vi "Periodic Tasks.vi"(11 "Initalizer":bool) -> ()   [LabVIEW 2014]
doc: "This VI runs in parallel to other tasks. It can contain as many user-defined periodic loops as you need. These can carry out PID or other sorts of timed response."
uses:
  <vilib>/Rock Robotics/SystemInterfaces/Utilities/FPGA_UtilitiesLED Source.ctl
  <vilib>/Rock Robotics/SystemInterfaces/Utilities/FPGA_UtilitiesLED State.ctl
  <vilib>/Rock Robotics/WPI/DriverStation/WPI_DriverStationRobotMode2.ctl
  Robot Global Data.vi
panel:
  in  "Skip Time":dbl=350.0
  in  "Loader Wait (ms)":u32=500
  in  "Wait Time (ms)":u32=500
  in  "Fire Time (ms)":u32=150
  in  "Min. Power":dbl=0.1 format="%#_13g"
  in  "Tolerance":dbl=1.0
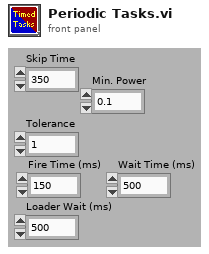
[diagram p1: front panel]
types:
  T1 = typedef "FPGA_UtilitiesLED State.ctl" = enum16{"Off", "On", "Toggle"}
  T2 = typedef "FPGA_UtilitiesLED Source.ctl" = enum16{"User LED", "FPGA LED"}
  T3 = cluster{"FIRE!!!":bool, "Loader":bool, "Lock":bool, "Load":bool, "Pass":bool, "Grab":bool, "PANIC":bool, "Don't Cock":bool, "Roller Speed":dbl}
  T4 = cluster{"Left Power":dbl, "Right Power":dbl, "Shooter State":enum16{"Nothing", "Fire", "Load"}, "Loader State":enum16{"Loader Up", "Loader Down", "Ball In Possesion"}, "Auto Time":dbl, "Tele Time":dbl, "Driver":dbl, "Not Allowed":bool, "Right Speed":dbl, "Left Speed":dbl}
  T5 = enum16{"Nothing", "Load", "Lock", "Pass", "Grab", "Loader Down", "Shoot", "Auto Start", "Tele Start"}
  T6 = typedef "WPI_DriverStationRobotMode2.ctl" = enum16{"Autonomous Disabled", "Autonomous Enabled", "Teleop Disabled", "Teleop Enabled", "Disconnected", "Finish", "Test Disabled", "Test Enabled"}
  T7 = enum16{"Nothing", "Loader Down", "Loader Up", "Load", "Grab", "Pass", "Fire", "Lock"}
  T8 = enum16{"Loader Up", "Loader Down", "Ball In Possesion"}
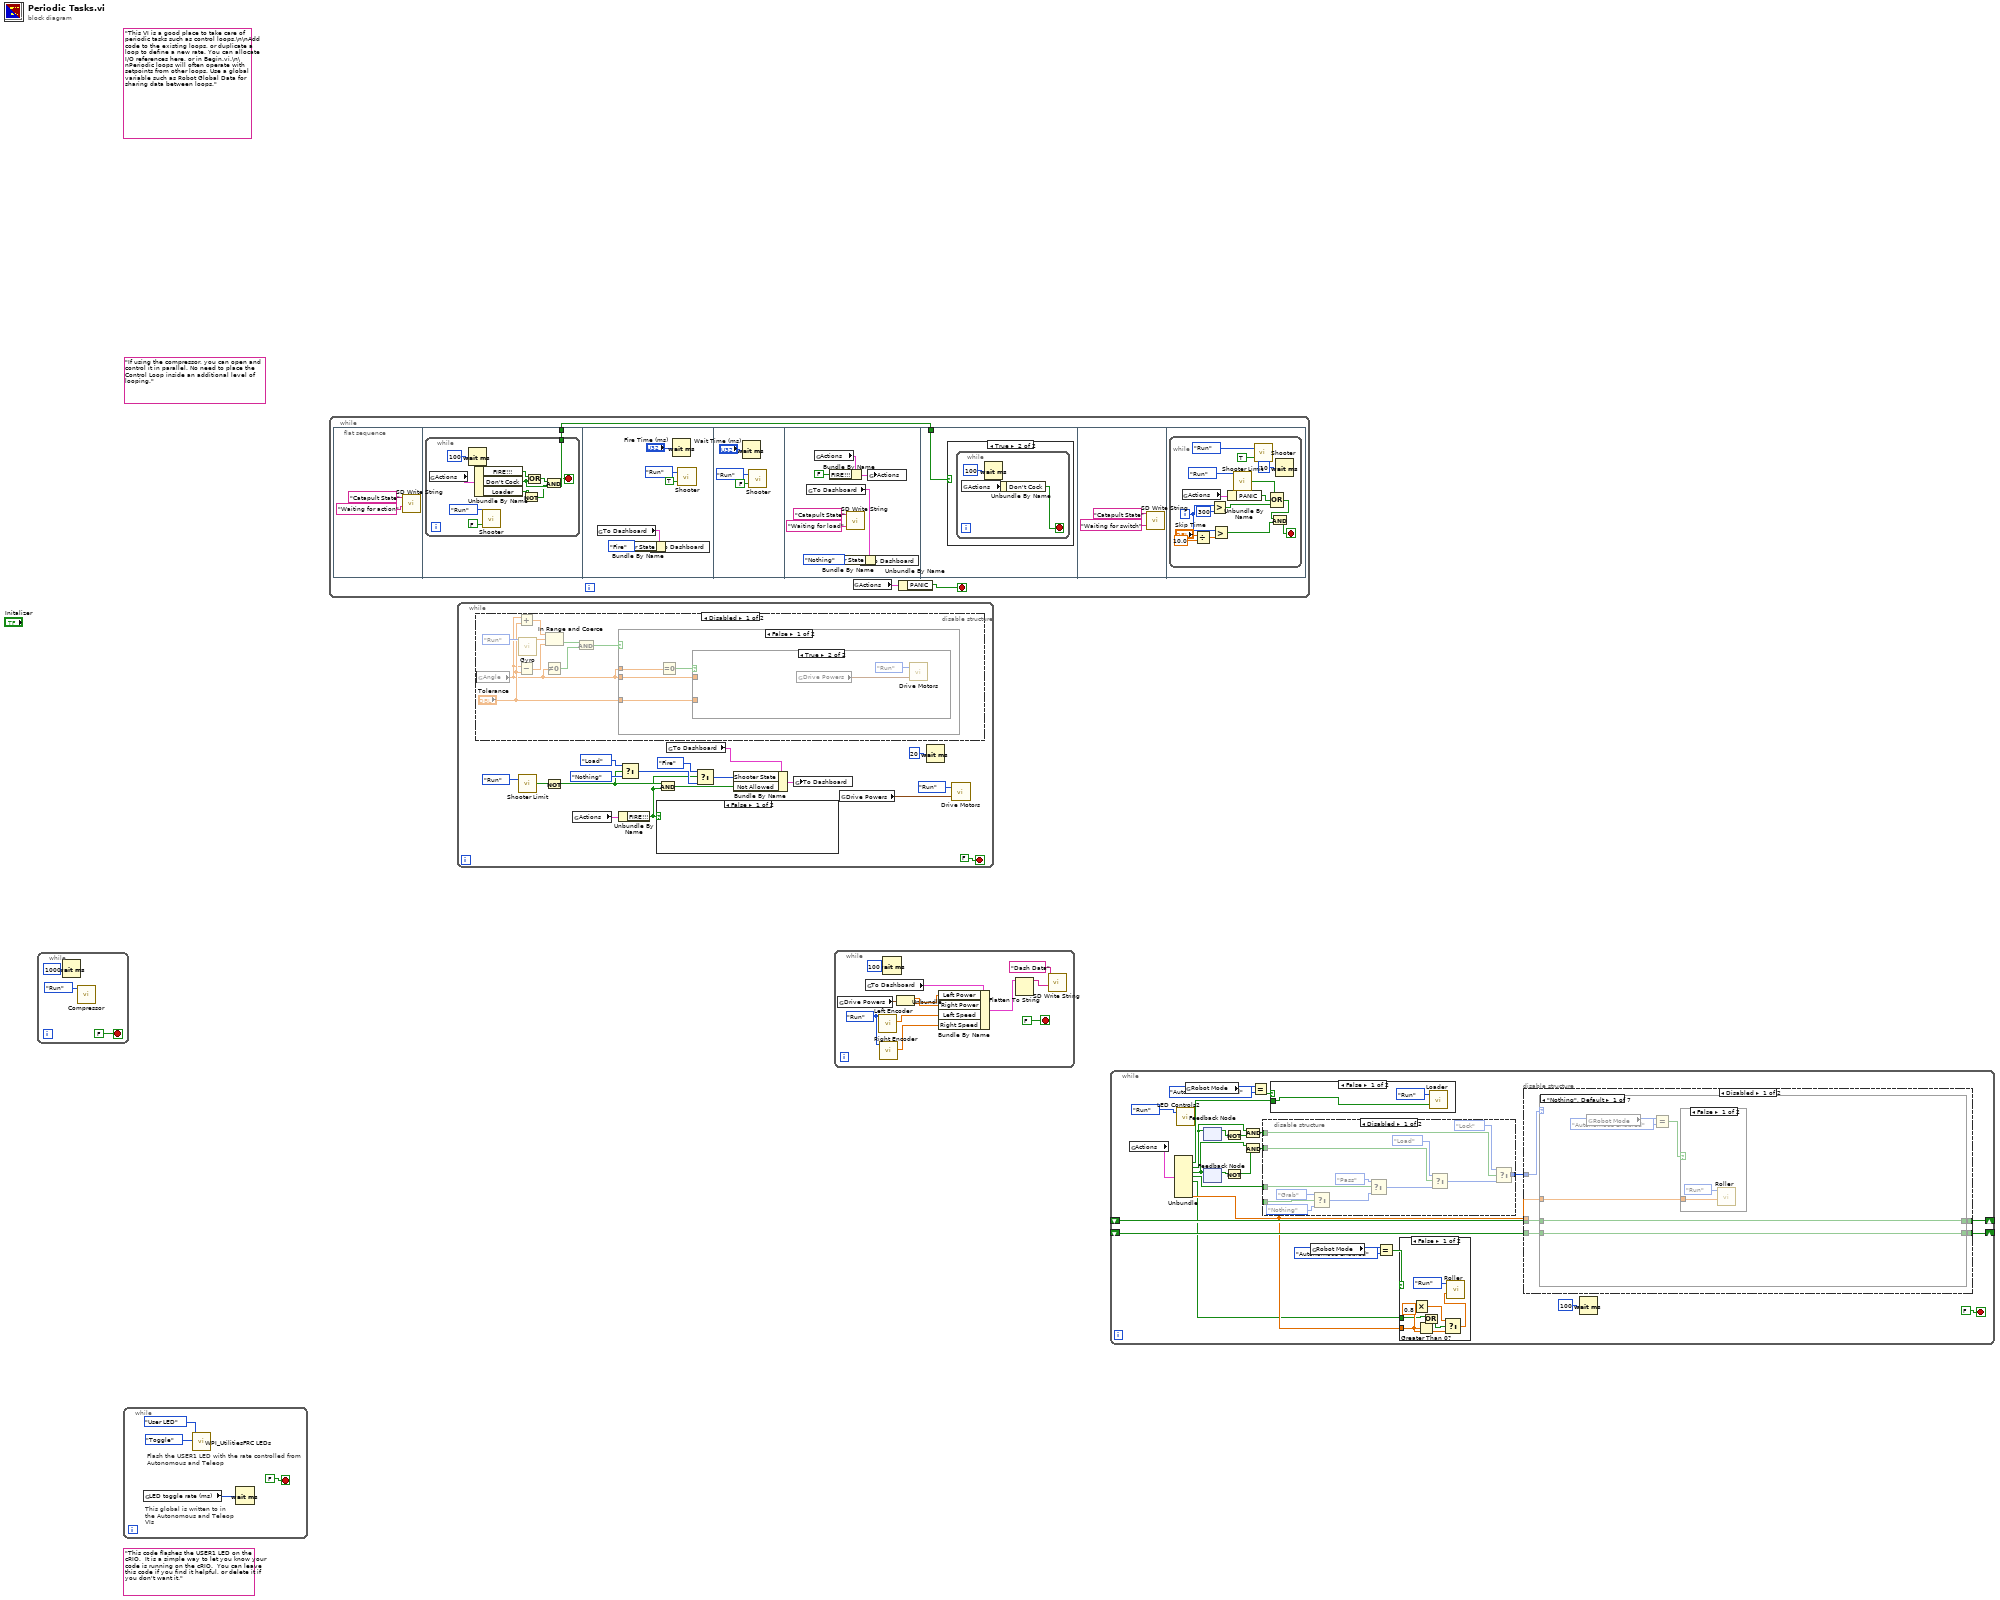
[diagram p0: block diagram]
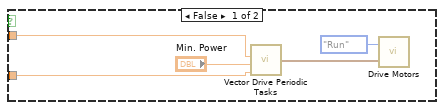
[diagram p3: hidden frame]
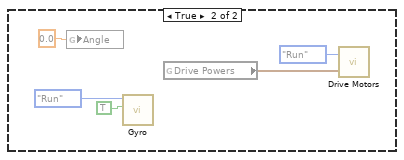
[diagram p4: hidden frame]
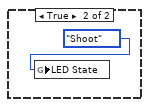
[diagram p6: hidden frame]
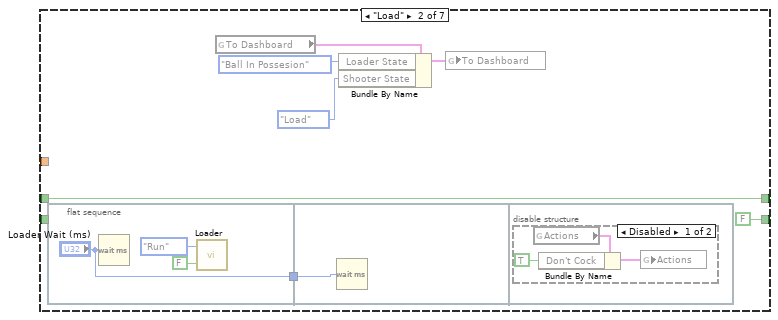
[diagram p9: hidden frame]
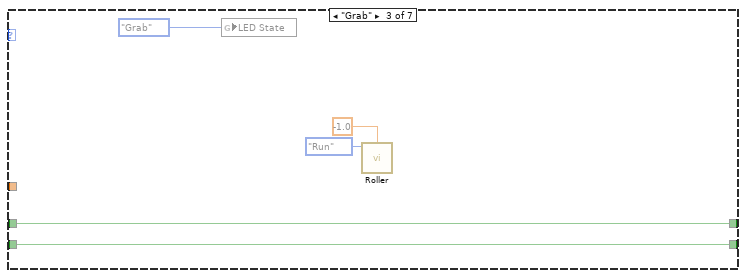
[diagram p11: hidden frame]
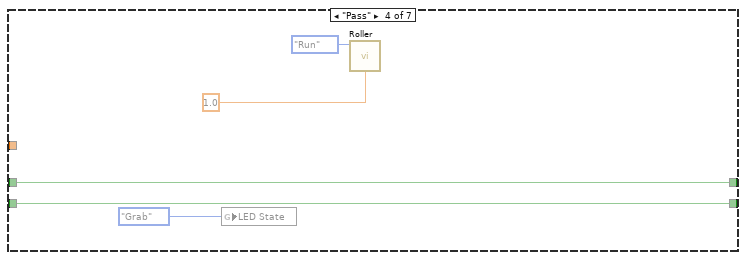
[diagram p12: hidden frame]
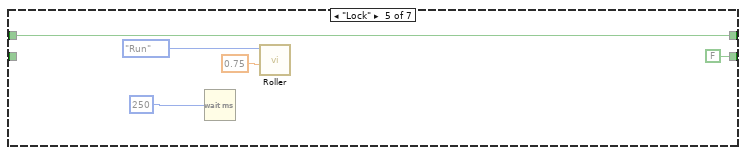
[diagram p13: hidden frame]
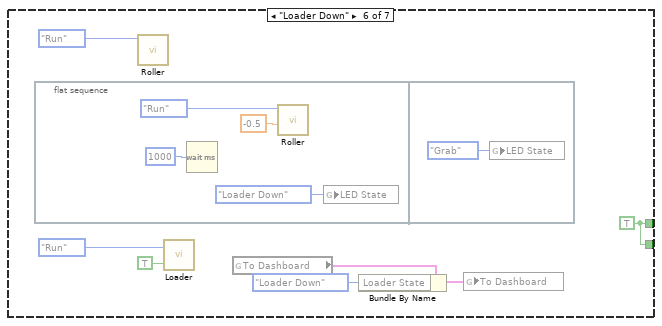
[diagram p14: hidden frame]
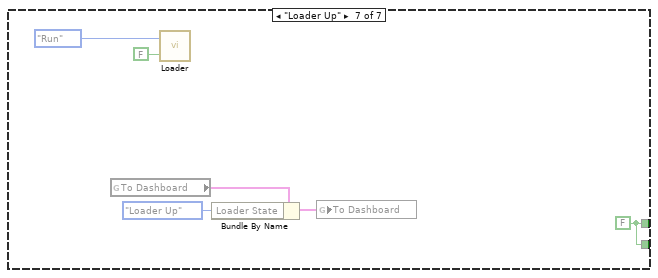
[diagram p15: hidden frame]
diagram:
  (unwired) "If using the compressor, you can open and control it in parallel. No need to place the Control Loop inside an additional level of looping."
  (unwired) "This code flashes the USER1 LED on the cRIO.  It is a simple way to let you know your code is running on the cRIO.  You can leave this code if you find it helpful, or delete it if you don't want it."
  (unwired) "This VI is a good place to take care of periodic tasks such as control loops.\n\nAdd code to the existing loops, or duplicate a loop to define a new rate. You can allocate I/O references here, or in Begin.vi.\n\nPeriodic loops will often operate with setpoints from other loops. Use a global variable such as Robot Global Data for sharing data between loops."
  n1 = while {
    stop <- FALSE stop-if-true
    n2 = Wait (ms)(milliseconds to wait=u32 1000) -> ()  [unwired: 1 out]
    n3 = call "Compressor.vi"("Enum"=enum16{"Start", "Run", "End"}."Run") -> ()  [unwired: 11 in]
  }
  n4 = while {
    stop <- FALSE stop-if-true
    # "This global is written to in the Autonomous and Teleop VIs"
    # "Flash the USER1 LED with the rate controlled from Autonomous and Teleop"
    n5 = global read "Robot Global Data.vi" "LED toggle rate (ms)"() -> (w4:u32)
    n6 = call <vilib>:"WPI_UtilitiesFRC LEDs.vi"("State"=FPGA_UtilitiesLED_State."Toggle", "LED Type"=FPGA_UtilitiesLED_Source."User LED") -> ()  [unwired: 1 in, 9 out]
    n7 = Wait (ms)(milliseconds to wait=w4) -> ()  [unwired: 1 out]
  }
  n8 = while {
    stop <- w9 stop-if-true
    n9 = flat-sequence {
      tunnel: [w13] -> w8
      tunnel: w8 -> [w41]
      frame #0 {
        n10 = call <vilib>:"SD Write String.vi"("String"="Waiting for action", "Name"="Catapult State") -> ()  [unwired: 8 in, 2 out]
      }
      frame #1 {
        n11 = while {
          tunnel: [w18] -> w13
          stop <- w16 stop-if-true
          n12 = global read "Robot Global Data.vi" "Actions"() -> (w23:T3)
          n13 = Wait (ms)(milliseconds to wait=u32 100) -> ()  [unwired: 1 out]
          n14 = Unbundle By Name(w23) -> ("FIRE!!!"=w19:bool, "Don't Cock"=w18:bool, "Loader"=w14:bool)
          n15 = call "Shooter.vi"("Run"=FALSE, "Enum"=enum16{"Start", "Run", "End"}."Run") -> ()  [unwired: 1 in]
          n16 = Not(x=w14) -> (.not. x?=w15:bool)
          n17 = Or(x=w19, y=w18) -> (x .or. y?=w17:bool)
          n18 = And(x=w17, y=w15) -> (x .and. y?=w16:bool)
        }
      }
      frame #2 {
        n19 = global read "Robot Global Data.vi" "To Dashboard"() -> (w25:T4)
        n20 = Bundle By Name(cluster=w25, "Shooter State"=enum16{"Nothing", "Fire", "Load"}."Fire") -> (w26:T4)
        n21 = global write "Robot Global Data.vi" "To Dashboard"(w26) -> ()
        n22 = Wait (ms)(milliseconds to wait="Fire Time (ms)") -> ()  [unwired: 1 out]
        n23 = call "Shooter.vi"("Run"=TRUE, "Enum"=enum16{"Start", "Run", "End"}."Run") -> ()  [unwired: 1 in]
      }
      frame #3 {
        n24 = Wait (ms)(milliseconds to wait="Wait Time (ms)") -> ()  [unwired: 1 out]
        n25 = call "Shooter.vi"("Run"=FALSE, "Enum"=enum16{"Start", "Run", "End"}."Run") -> ()  [unwired: 1 in]
      }
      frame #4 {
        n26 = global read "Robot Global Data.vi" "To Dashboard"() -> (w36:T4)
        n27 = global read "Robot Global Data.vi" "Actions"() -> (w38:T3)
        n28 = Bundle By Name(cluster=w36, "Shooter State"=enum16{"Nothing", "Fire", "Load"}."Nothing") -> (w37:T4)
        n29 = Bundle By Name(cluster=w38, "FIRE!!!"=FALSE) -> (w40:T3)
        n30 = call <vilib>:"SD Write String.vi"("String"="Waiting for load", "Name"="Catapult State") -> ()  [unwired: 8 in, 2 out]
        n31 = global write "Robot Global Data.vi" "To Dashboard"(w37) -> ()
        n32 = global write "Robot Global Data.vi" "Actions"(w40) -> ()
      }
      frame #5 {
        n33 = case shown="True" w41 {
          frame False {
          }
          frame True {
            n34 = while {
              stop <- w42 stop-if-true
              n35 = global read "Robot Global Data.vi" "Actions"() -> (w44:T3)
              n36 = Wait (ms)(milliseconds to wait=u32 100) -> ()  [unwired: 1 out]
              n37 = Unbundle By Name(w44) -> ("Don't Cock"=w42:bool)
            }
          }
        }
      }
      frame #6 {
        n38 = call <vilib>:"SD Write String.vi"("String"="Waiting for switch", "Name"="Catapult State") -> ()  [unwired: 8 in, 2 out]
      }
      frame #7 {
        n39 = while {
          i -> [w51]
          stop <- w53 stop-if-true
          n40 = global read "Robot Global Data.vi" "Actions"() -> (w58:T3)
          n41 = Divide(x="Skip Time", y=10.0) -> (x/y=w47:dbl)
          n42 = Greater?(x=w51, y=300) -> (0:w54:bool)
          n43 = Greater?(x=w51, y=w47) -> (0:w50:bool)
          n44 = Unbundle By Name(w58) -> ("PANIC"=w57:bool)
          n45 = call "Shooter Limit.vi"("Enum"=enum16{"Start", "Run", "End"}."Run") -> ("Value"=w56:bool)  [unwired: 1 in]
          n46 = call "Shooter.vi"("Run"=TRUE, "Enum"=enum16{"Start", "Run", "End"}."Run") -> ()  [unwired: 1 in]
          n47 = Compound Arithmetic op=OR(w56, w57, w54) -> (w52:bool)
          n48 = And(x=w52, y=w50) -> (x .and. y?=w53:bool)
          n49 = Wait (ms)(milliseconds to wait=u32 10) -> ()  [unwired: 1 out]
        }
      }
    }
    n50 = global read "Robot Global Data.vi" "Actions"() -> (w10:T3)
    n51 = Unbundle By Name(w10) -> ("PANIC"=w9:bool)
  }
  n52 = while {
    stop <- FALSE stop-if-true
    n53 = disable-structure shown="Disabled" {
      frame Disabled {
        n54 = global read "Robot Global Data.vi" "Angle"() -> (w80:dbl)
        n55 = Add(x=w80, y="Tolerance") -> (x+y=w88:dbl)
        n56 = Subtract(x=w80, y="Tolerance") -> (x-y=w87:dbl)
        n57 = call "Gyro.vi"("Enum"=enum16{"Start", "Run", "End"}."Run") -> ("Angle"=w85:dbl)  [unwired: 10 in]
        n58 = Not Equal To 0?(x=w80) -> (x != 0?=w82:bool)
        n59 = In Range and Coerce(upper limit=w88, x=w85, lower limit=w87) -> (In Range?=w81:bool)  [unwired: 1 out]
        n60 = And(x=w81, y=w82) -> (x .and. y?=w83:bool)
        n61 = case shown="False" w83 {
          tunnel: w80 -> [w92 _]
          tunnel: "Tolerance" -> [w91 _]
          tunnel: w80 -> [w90 _]
          frame False {
            n62 = Equal To 0?(x=w92) -> (x = 0?=w89:bool)
            n63 = case shown="True" w89 {
              tunnel: w91 -> [w96 _]
              tunnel: w90 -> [w93 _]
              frame False {
                n64 = call "Vector Drive Periodic Tasks.vi"("Tolerance"=w96, "Min. Power"="Min. Power", "Angle"=w93) -> ("Motor Powers"=w94:cluster{"RMotor":dbl, "LMotor":dbl})  [unwired: 1 in]
                n65 = call "Drive Motors.vi"("Motor Powers"=w94, "Enum"=enum16{"Start", "Run", "End"}."Run") -> ()
              }
              frame True {
                n66 = global read "Robot Global Data.vi" "Drive Powers"() -> (w99:cluster{"Right":dbl, "Left":dbl})
                n67 = call "Drive Motors.vi"("Motor Powers"=w99, "Enum"=enum16{"Start", "Run", "End"}."Run") -> ()
              }
            }
          }
          frame True {
            n68 = global write "Robot Global Data.vi" "Angle"(0.0 ("Angle")) -> ()
            n69 = call "Gyro.vi"("Reset"=TRUE, "Enum"=enum16{"Start", "Run", "End"}."Run") -> ()  [unwired: 9 in, 1 out]
            n70 = global read "Robot Global Data.vi" "Drive Powers"() -> (w101:cluster{"Right":dbl, "Left":dbl})
            n71 = call "Drive Motors.vi"("Motor Powers"=w101, "Enum"=enum16{"Start", "Run", "End"}."Run") -> ()
          }
        }
      }
      frame Enabled {
      }
    }
    n72 = call "Shooter Limit.vi"("Enum"=enum16{"Start", "Run", "End"}."Run") -> ("Value"=w77:bool)  [unwired: 1 in]
    n73 = Not(x=w77) -> (.not. x?=w67:bool)
    n74 = global read "Robot Global Data.vi" "Actions"() -> (w66:T3)
    n75 = Unbundle By Name(w66) -> ("FIRE!!!"=w65:bool)
    n76 = Select(t=enum16{"Nothing", "Fire", "Load"}."Load" ("Shooter State"), s=w67, f=enum16{"Nothing", "Fire", "Load"}."Nothing" ("Shooter State")) -> (s? t:f=w70:enum16{"Nothing", "Fire", "Load"})
    n77 = case shown="False" w65 {
      frame False {
      }
      frame True {
        n78 = global write "Robot Global Data.vi" "LED State"(T5."Shoot" ("LED State")) -> ()
      }
    }
    n79 = And(x=w67, y=w65) -> (x .and. y?=w68:bool)
    n80 = global read "Robot Global Data.vi" "To Dashboard"() -> (w75:T4)
    n81 = Select(t=enum16{"Nothing", "Fire", "Load"}."Fire" ("Shooter State"), s=w65, f=w70) -> (s? t:f=w74:enum16{"Nothing", "Fire", "Load"})
    n82 = Bundle By Name(cluster=w75, "Shooter State"=w74, "Not Allowed"=w68) -> (w69:T4)
    n83 = global write "Robot Global Data.vi" "To Dashboard"(w69) -> ()
    n84 = global read "Robot Global Data.vi" "Drive Powers"() -> (w63:cluster{"Right":dbl, "Left":dbl})
    n85 = Wait (ms)(milliseconds to wait=u32 20) -> ()  [unwired: 1 out]
    n86 = call "Drive Motors.vi"("Motor Powers"=w63, "Enum"=enum16{"Start", "Run", "End"}."Run") -> ()
  }
  n87 = while {
    stop <- FALSE stop-if-true
    w109 = enum16{"Start", "Run", "End"}."Run" ("Enum")
    n88 = global read "Robot Global Data.vi" "Drive Powers"() -> (w114:cluster{"Right":dbl, "Left":dbl})
    n89 = global read "Robot Global Data.vi" "To Dashboard"() -> (w115:T4)
    n90 = call "Left Encoder.vi"("Enum"=w109) -> ("Rate"=w108:dbl)  [unwired: 9 in, 1 out]
    n91 = call "Right Encoder.vi"("Enum"=w109) -> ("Rate"=w107:dbl)  [unwired: 9 in, 1 out]
    n92 = Wait (ms)(milliseconds to wait=u32 100) -> ()  [unwired: 1 out]
    n93 = Unbundle(w114) -> ("Right"=w113:dbl, "Left"=w112:dbl)
    n94 = Bundle By Name(cluster=w115, "Left Power"=w112, "Right Power"=w113, "Left Speed"=w108, "Right Speed"=w107) -> (w111:T4)
    n95 = Flatten To String(anything=w111) -> (data string=w106:string)  [unwired: 3 in, 2 out]
    n96 = call <vilib>:"SD Write String.vi"("String"=w106, "Name"="Dash Data") -> ()  [unwired: 8 in, 2 out]
  }
  n97 = while {
    shift-right: [w142] -> _
    shift-left: _ -> [w140]
    shift-right: [w131] -> _
    shift-left: _ -> [w130]
    stop <- FALSE stop-if-true
    n98 = global read "Robot Global Data.vi" "Actions"() -> (w141:T3)
    n99 = Unbundle(w141) -> ("Loader"=w127:bool, "Lock"=w136:bool, "Load"=w132:bool, "Pass"=w129:bool, "Grab"=w118:bool, "Roller Speed"=w120:dbl)  [unwired: 3 out]
    n100 = call "LED Controls2.vi"("Enum"=enum16{"Start", "Run", "End"}."Run") -> ()  [unwired: 2 in]
    n101 = global read "Robot Global Data.vi" "Robot Mode"() -> (w125:T6)
    n102 = feedback #1() -> (w138:bool)  [unwired: 1 in]
    n103 = feedback-in #1(w136) -> ()
    n104 = feedback #2() -> (w135:bool)  [unwired: 1 in]
    n105 = feedback-in #2(w132) -> ()
    n106 = Not(x=w138) -> (.not. x?=w139:bool)
    n107 = Not(x=w135) -> (.not. x?=w134:bool)
    n108 = And(x=w136, y=w139) -> (x .and. y?=w137:bool)
    n109 = And(x=w132, y=w134) -> (x .and. y?=w133:bool)
    n110 = Equal?(x=w125, y=WPI_DriverStationRobotMode2."Autonomous Enabled") -> (x = y?=w124:bool)
    n111 = disable-structure shown="Disabled" {
      disable-tunnel: w137 -> [w152 _]
      disable-tunnel: w133 -> [w151 _]
      disable-tunnel: w129 -> [w147 _]
      disable-tunnel: _ -> [w146 _]
      disable-tunnel: [w145 _] -> w128
      frame Disabled {
        n112 = Select(t=T7."Grab", s=w146, f=T7."Nothing" ("Loader State")) -> (s? t:f=w149:T7)
        n113 = Select(t=T7."Pass" ("Loader State"), s=w147, f=w149) -> (s? t:f=w154:T7)
        n114 = Select(t=T7."Load" ("Loader State"), s=w151, f=w154) -> (s? t:f=w156:T7)
        n115 = Select(t=T7."Lock" ("Loader State"), s=w152, f=w156) -> (s? t:f=w145:T7)
      }
      frame Enabled {
      }
    }
    n116 = case shown="False" w124 {
      tunnel: w127 -> [w227 _]
      frame False {
        n117 = call "Loader.vi"("Down (Forward)"=w227, "Enum"=enum16{"Start", "Run", "End"}."Run") -> ()  [unwired: 1 out]
      }
      frame True {
      }
    }
    n118 = global read "Robot Global Data.vi" "Robot Mode"() -> (w121:T6)
    n119 = Equal?(x=w121, y=WPI_DriverStationRobotMode2."Autonomous Enabled") -> (x = y?=w123:bool)
    n120 = case shown="False" w123 {
      tunnel: w120 -> [w224 _]
      tunnel: w118 -> [w219 _]
      frame False {
        n121 = Multiply(x=w224, y=0.8) -> (x*y=w222:dbl)
        n122 = Greater Than 0?(x=w224) -> (x > 0?=w221:bool)
        n123 = Or(x=w219, y=w221) -> (x .or. y?=w220:bool)
        n124 = Select(t=w222, s=w220, f=w224) -> (s? t:f=w225:dbl)
        n125 = call "Roller.vi"("Power"=w225, "Enum"=enum16{"Start", "Run", "End"}."Run") -> ()  [unwired: 2 in]
      }
      frame True {
      }
    }
    n126 = disable-structure shown="Disabled" {
      disable-tunnel: [w163 _] -> w142
      disable-tunnel: w140 -> [w162 _]
      disable-tunnel: [w161 _] -> w131
      disable-tunnel: w130 -> [w160 _]
      disable-tunnel: w128 -> [w159 _]
      disable-tunnel: w120 -> [w158 _]
      frame Disabled {
        n127 = case shown="\"Nothing\", Default" w159 {
          tunnel: [w169 w178 w189 w192 w197 w204 w216] -> w163
          tunnel: w162 -> [w169 w178 w189 w192 w197 _ _]
          tunnel: [w168 FALSE ("Down (Forward)") w186 w191 FALSE ("Down (Forward)") w204 w216] -> w161
          tunnel: w160 -> [w168 _ w186 w191 _ _ _]
          tunnel: w158 -> [w164 _ _ _ _ _ _]
          frame "Nothing", Default {
            n128 = global read "Robot Global Data.vi" "Robot Mode"() -> (w167:T6)
            n129 = Equal?(x=w167, y=WPI_DriverStationRobotMode2."Autonomous Enabled") -> (x = y?=w165:bool)
            n130 = case shown="False" w165 {
              tunnel: w164 -> [w170 _]
              frame False {
                n131 = call "Roller.vi"("Power"=w170, "Enum"=enum16{"Start", "Run", "End"}."Run") -> ()  [unwired: 2 in]
              }
              frame True {
              }
            }
          }
          frame "Load" {
            n132 = flat-sequence {
              tunnel: ["Loader Wait (ms)"] -> w172
              tunnel: w172 -> [w182]
              frame #0 {
                n133 = Wait (ms)(milliseconds to wait="Loader Wait (ms)") -> ()  [unwired: 1 out]
                n134 = call "Loader.vi"("Down (Forward)"=FALSE, "Enum"=enum16{"Start", "Run", "End"}."Run") -> ()  [unwired: 1 out]
              }
              frame #1 {
                n135 = Wait (ms)(milliseconds to wait=w182) -> ()  [unwired: 1 out]
              }
              frame #2 {
                n136 = disable-structure shown="Disabled" {
                  frame Disabled {
                    n137 = global read "Robot Global Data.vi" "Actions"() -> (w185:T3)
                    n138 = Bundle By Name(cluster=w185, "Don't Cock"=TRUE) -> (w184:T3)
                    n139 = global write "Robot Global Data.vi" "Actions"(w184) -> ()
                  }
                  frame Enabled {
                  }
                }
              }
            }
            n140 = global read "Robot Global Data.vi" "To Dashboard"() -> (w176:T4)
            n141 = Bundle By Name(cluster=w176, "Loader State"=T8."Ball In Possesion", "Shooter State"=enum16{"Nothing", "Fire", "Load"}."Load") -> (w174:T4)
            n142 = global write "Robot Global Data.vi" "To Dashboard"(w174) -> ()
          }
          frame "Grab" {
            n143 = global write "Robot Global Data.vi" "LED State"(T5."Grab" ("LED State")) -> ()
            n144 = call "Roller.vi"("Power"=-1.0, "Enum"=enum16{"Start", "Run", "End"}."Run") -> ()  [unwired: 2 in]
          }
          frame "Pass" {
            n145 = global write "Robot Global Data.vi" "LED State"(T5."Grab" ("LED State")) -> ()
            n146 = call "Roller.vi"("Power"=1.0 ("Pass Power"), "Enum"=enum16{"Start", "Run", "End"}."Run") -> ()  [unwired: 2 in]
          }
          frame "Lock" {
            n147 = Wait (ms)(milliseconds to wait=u32 250) -> ()  [unwired: 1 out]
            n148 = call "Roller.vi"("Power"=0.75, "Enum"=enum16{"Start", "Run", "End"}."Run") -> ()  [unwired: 2 in]
          }
          frame "Loader Down" {
            w204 = TRUE ("Down (Forward)")
            n149 = flat-sequence {
              frame #0 {
                n150 = Wait (ms)(milliseconds to wait=u32 1000) -> ()  [unwired: 1 out]
                n151 = call "Roller.vi"("Power"=-0.5, "Enum"=enum16{"Start", "Run", "End"}."Run") -> ()  [unwired: 2 in]
                n152 = global write "Robot Global Data.vi" "LED State"(T5."Loader Down" ("LED State")) -> ()
              }
              frame #1 {
                n153 = global write "Robot Global Data.vi" "LED State"(T5."Grab" ("LED State")) -> ()
              }
            }
            n154 = call "Roller.vi"("Enum"=enum16{"Start", "Run", "End"}."Run") -> ()  [unwired: 3 in]
            n155 = call "Loader.vi"("Down (Forward)"=TRUE, "Enum"=enum16{"Start", "Run", "End"}."Run") -> ()  [unwired: 1 out]
            n156 = global read "Robot Global Data.vi" "To Dashboard"() -> (w203:T4)
            n157 = Bundle By Name(cluster=w203, "Loader State"=T8."Loader Down") -> (w201:T4)
            n158 = global write "Robot Global Data.vi" "To Dashboard"(w201) -> ()
          }
          frame "Loader Up" {
            w216 = FALSE
            n159 = global read "Robot Global Data.vi" "To Dashboard"() -> (w215:T4)
            n160 = call "Loader.vi"("Down (Forward)"=FALSE, "Enum"=enum16{"Start", "Run", "End"}."Run") -> ()  [unwired: 1 out]
            n161 = Bundle By Name(cluster=w215, "Loader State"=T8."Loader Up") -> (w213:T4)
            n162 = global write "Robot Global Data.vi" "To Dashboard"(w213) -> ()
          }
        }
      }
      frame Enabled {
      }
    }
    n163 = Wait (ms)(milliseconds to wait=u32 100) -> ()  [unwired: 1 out]
  }
